vi "FPGA UART.vi"(0 "Clock Frequency":u32=120000000, 1 "Tx IO":refnum<k21>="IO Module\\TTL Out 2", 2 "Rx IO":refnum<k21>="IO Module\\TTL In 3", 5 "Baud Rate":u32=250000, 7 "Data Bits":u8=8 min=5 max=8 step=1, 9 "Stop Bit":u8=1, 11 "Invert Polarity?":bool=TRUE, 12 "Input Valid?":bool, 13 "Tx Data":u8) -> (4 "Rx Data":u8, 6 "Data Received?":bool, 15 "Ready for Input?":bool)   [LabVIEW 2015]
uses:
  Tick Counts.ctl
  Rx States.ctl
  Tx States.ctl
  <vilib>/rvi/FXPMathLib/FxpDiv/subVIs/nifxpmath_Div_SimConfig.ctl
  <vilib>/rvi/Emulation/niFpgaSctlEmulationGetInTimedLoop.vi
  <vilib>/rvi/Emulation/niFpgaProcessEmulError.vi
  <vilib>/rvi/eio/common/nirviEmuTemplateMethod_errors.vi
  <vilib>/rvi/FXPMathLib/FxpDiv/simVIs/DllFxpDivTemp_sub.vi
  <vilib>/eio/EIONode/EIONode.xnode
  <vilib>/rvi/FXPMathLib/FxpDiv/XNode/nifxpmath_Div.xnode
panel:
  out "Tick Counts":T1
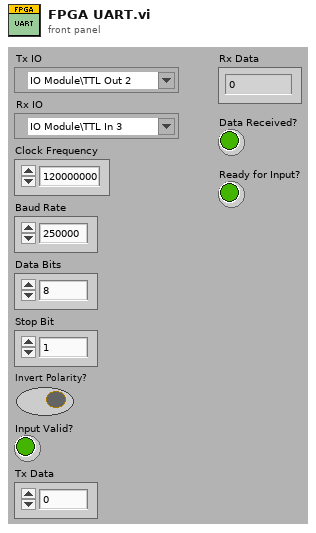
[diagram p1: front panel]
types:
  T1 = typedef "Tick Counts.ctl" = cluster{"Half Bit":u32, "One Bit":u32, "One and Half Bit":u32, "Two Bit":u32}
  T2 = typedef "Tx States.ctl" = enum16{"Wait for Input", "Send Start Bit", "Wait Start", "Send Data Bits", "Wait Send", "Send Parity Bit", "Wait Parity", "Send Stop Bit", "Wait 1 Bit", "Wait 1.5 Bit", "Wait 2 Bit"}
  T3 = typedef "Rx States.ctl" = enum16{"Wait for Start", "Wait Start", "Wait Receive", "Receive Data Bits", "Receive Parity Bit", "Wait Parity", "Wait 1 Bit", "Wait 1.5 Bit", "Wait 2 Bit", "Transfer Rx Data"}
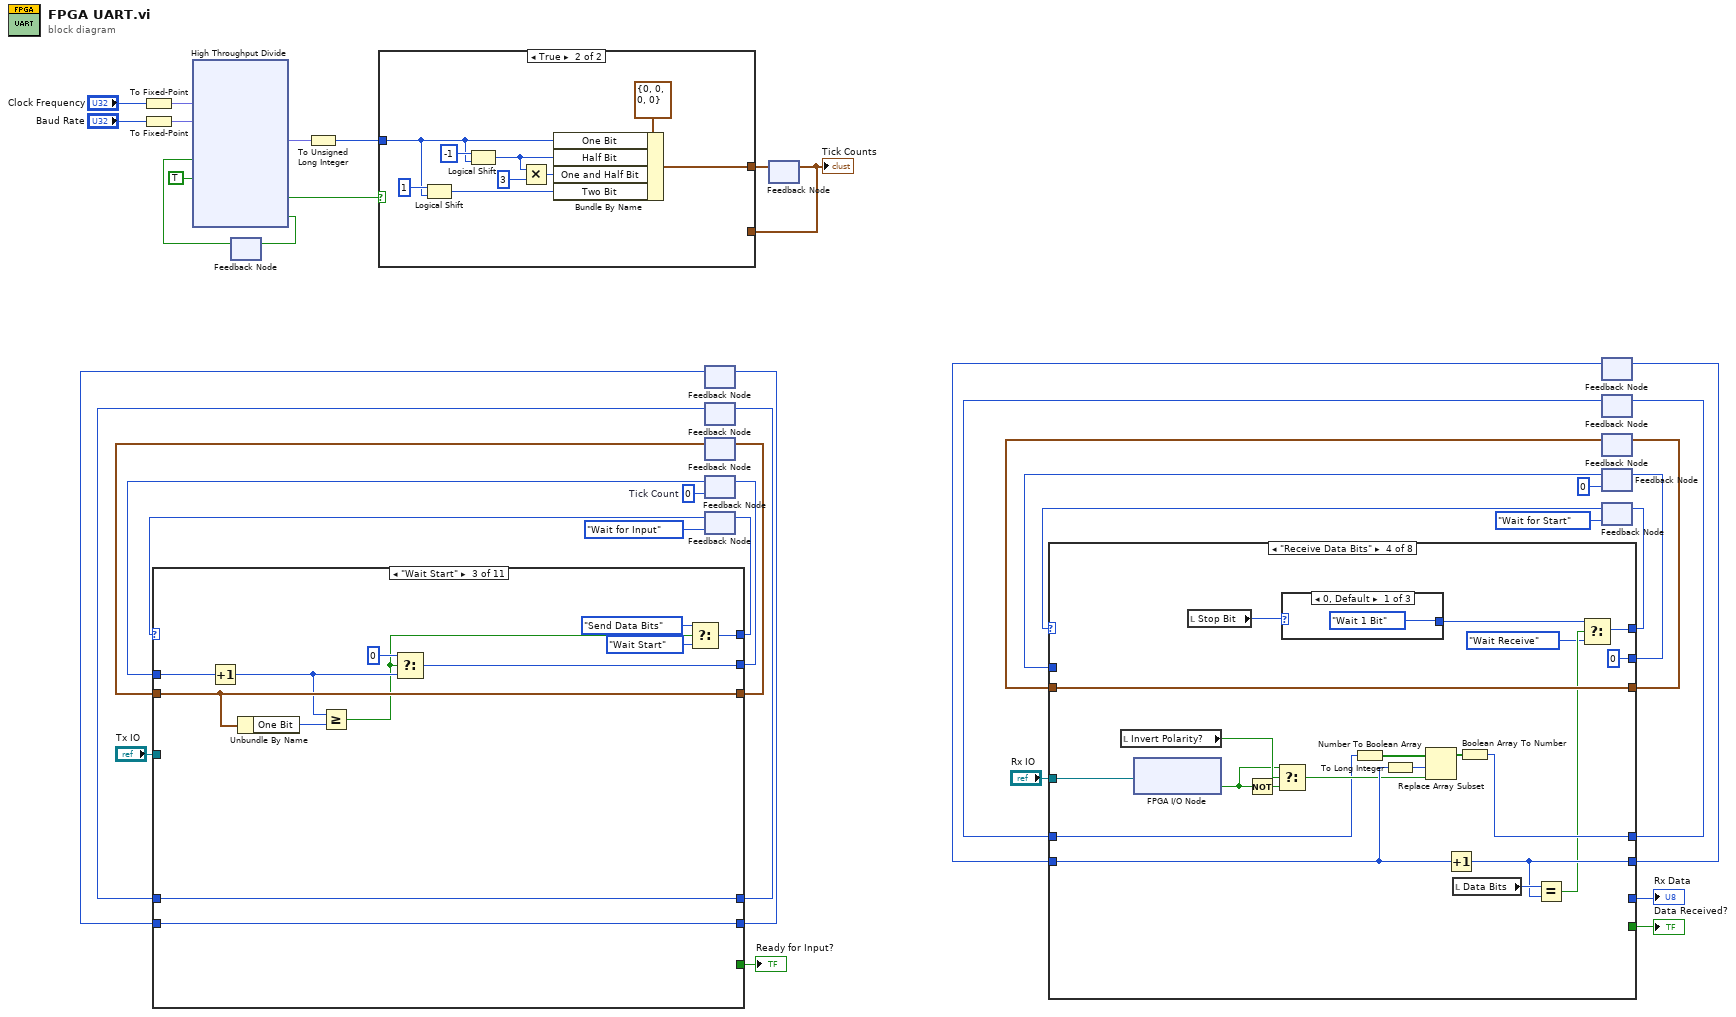
[diagram p0: block diagram]
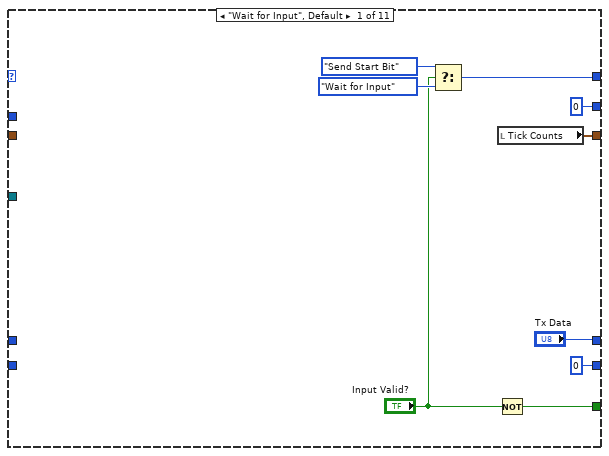
[diagram p2: hidden frame]
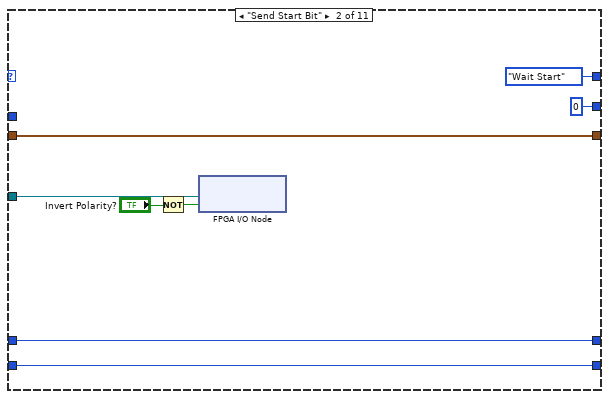
[diagram p3: hidden frame]
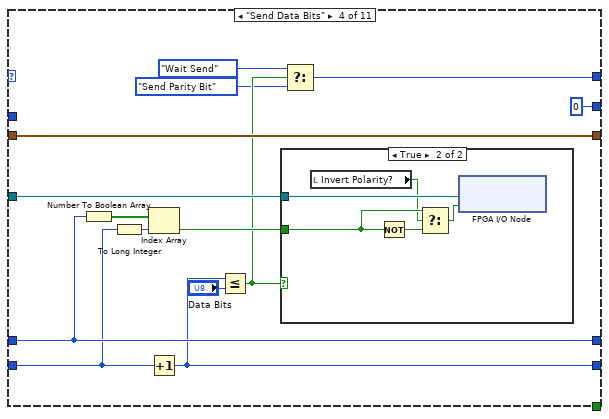
[diagram p4: hidden frame]
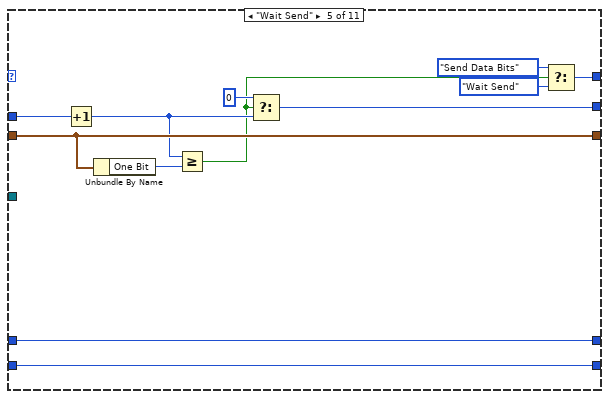
[diagram p6: hidden frame]
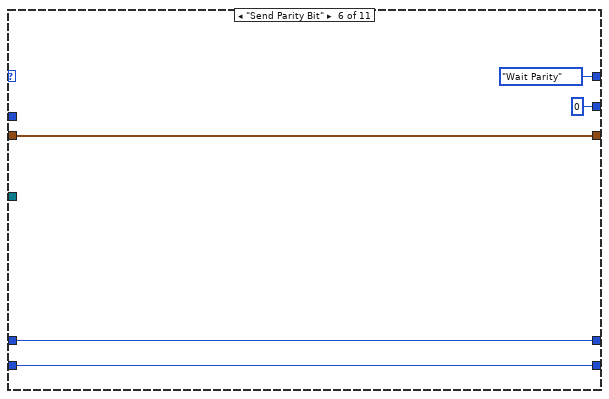
[diagram p7: hidden frame]
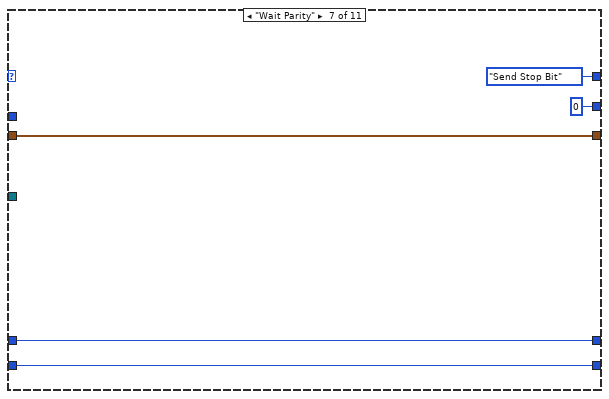
[diagram p8: hidden frame]
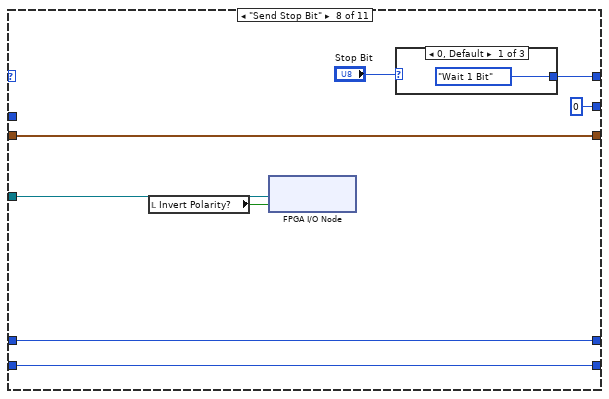
[diagram p9: hidden frame]
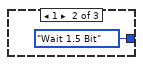
[diagram p10: hidden frame]
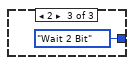
[diagram p11: hidden frame]
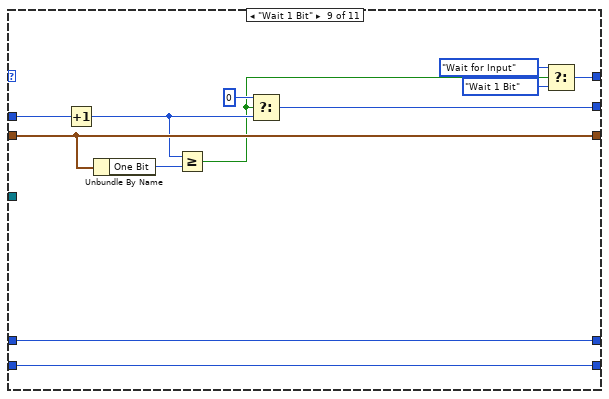
[diagram p12: hidden frame]
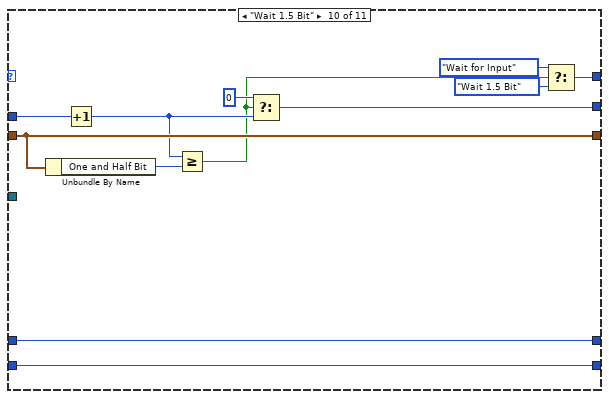
[diagram p13: hidden frame]
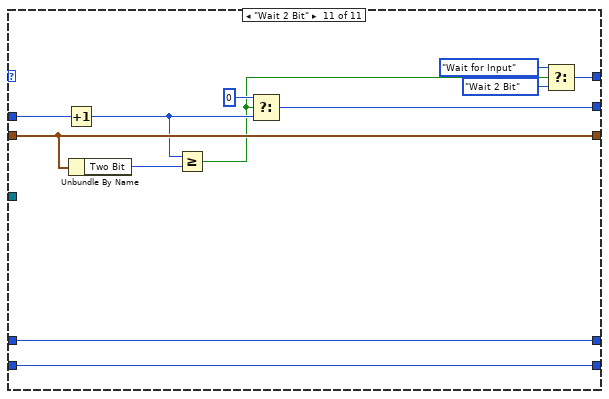
[diagram p14: hidden frame]
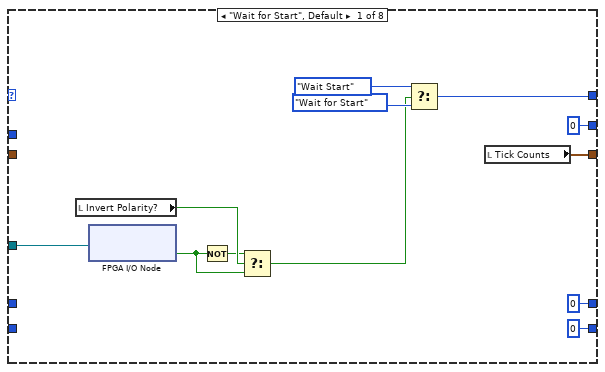
[diagram p15: hidden frame]
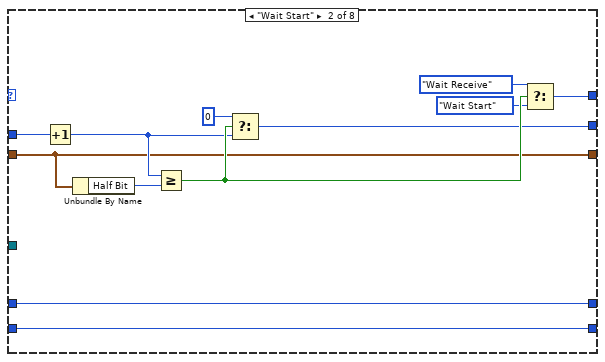
[diagram p16: hidden frame]
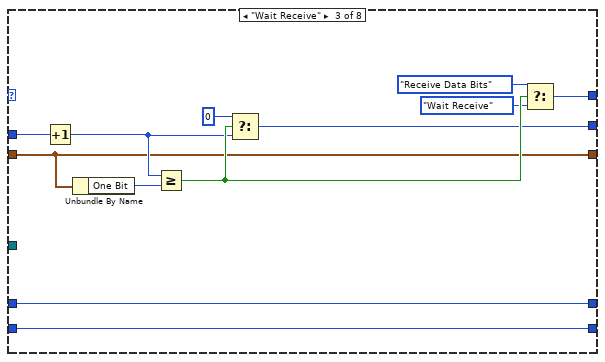
[diagram p17: hidden frame]
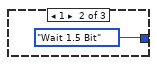
[diagram p18: hidden frame]
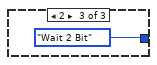
[diagram p19: hidden frame]
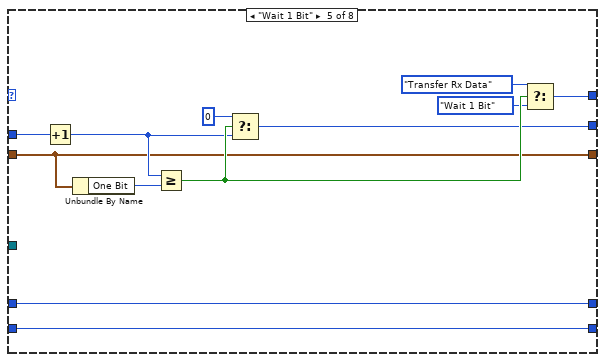
[diagram p20: hidden frame]
diagram:
  w9 = u32 0  # Tick Count
  n1 = To Fixed-Point(number="Clock Frequency") -> (fixed-point=w39:fxp<+,32,32>)  [unwired: 1 in]
  n2 = To Fixed-Point(number="Baud Rate") -> (fixed-point=w38:fxp<+,32,32>)  [unwired: 1 in]
  n3 = feedback #1() -> (w36:bool)  [unwired: 1 in]
  n4 = xnode "High Throughput Divide"("x"=w39, "y"=w38, "input valid"=w36, "ready for output (T)"=TRUE) -> ("x/y"=w33:fxp<+,32,32>, "output valid"=w34:bool, "ready for input"=w37:bool)
  n5 = feedback-in #1(w37) -> ()
  n6 = To Unsigned Long Integer(number=w33) -> (unsigned 32bit integer=w32:u32)
  n7 = feedback #2() -> (w5:u8)  [unwired: 1 in]
  n8 = feedback #3() -> (w7:u8)  [unwired: 1 in]
  n9 = feedback #4() -> (w4:T1)  [unwired: 1 in]
  n10 = feedback #5(w9) -> (w10:u32)
  n11 = feedback #6(Tx_States."Wait for Input" ("Enum")) -> (w13:T2)
  n12 = case shown="\"Wait Start\"" w13 {
    tunnel: [w45 Tx_States."Wait Start" ("Enum") w64 w73 w95 Tx_States."Wait Parity" ("Enum") Tx_States."Send Stop Bit" ("Enum") w113 w128 w140 w152] -> w14
    tunnel: ["Tx Data" w56 w60 w83 w91 w103 w107 w115 w124 w136 w148] -> w3
    tunnel: w7 -> [_ w56 w60 w83 w91 w103 w107 w115 w124 w136 w148]
    tunnel: "Tx IO" -> [_ w58 _ w76 _ _ _ w116 _ _ _]
    tunnel: w10 -> [_ _ w70 _ w101 _ _ _ w134 w146 w158]
    tunnel: [u32 0 u32 0 ("t") w66 u32 0 ("t") w97 u32 0 ("t") u32 0 ("t") u32 0 ("t") w130 w142 w154] -> w11
    tunnel: [w44 w54 w69 w81 w100 w106 w111 w119 w133 w145 w157] -> w8
    tunnel: w4 -> [_ w54 w69 w81 w100 w106 w111 w119 w133 w145 w157]
    tunnel: w5 -> [_ w52 w59 w80 w90 w105 w110 w118 w123 w135 w147]
    tunnel: [u8 0 ("Send Bit Count") w52 w59 w78 w90 w105 w110 w118 w123 w135 w147] -> w6
    tunnel: [w42 _ _ _ _ _ _ _ _ _ _] -> w2
    frame "Wait for Input", Default {
      n13 = Select(t=Tx_States."Send Start Bit", s="Input Valid?", f=Tx_States."Wait for Input" ("Enum")) -> (s? t:f=w45:T2)
      n14 = Not(x="Input Valid?") -> (.not. x?=w42:bool)
      n15 = local read "Tick Counts"() -> (w44:T1)
    }
    frame "Send Start Bit" {
      n16 = Not(x="Invert Polarity?") -> (.not. x?=w57:bool)
      n17 = xnode "FPGA I/O Node"("I/O Item"=w57, "FPGA I/O In"=w58) -> ()  [unwired: 1 out]
    }
    frame "Wait Start" {
      n18 = Increment(x=w70) -> (x+1=w67:u32)
      n19 = Unbundle By Name(w69) -> ("One Bit"=w68:u32)
      n20 = Greater Or Equal?(x=w67, y=w68) -> (x >= y?=w63:bool)
      n21 = Select(t=u32 0, s=w63, f=w67) -> (s? t:f=w66:u32)
      n22 = Select(t=Tx_States."Send Data Bits", s=w63, f=Tx_States."Wait Start" ("Enum")) -> (s? t:f=w64:T2)
    }
    frame "Send Data Bits" {
      n23 = Number To Boolean Array(number=w83) -> (Boolean array=w82:bool[])
      n24 = To Long Integer(number=w80) -> (32bit integer=w79:i32)
      n25 = Index Array(array=w82, index=w79) -> (element=w75:bool)
      n26 = Increment(x=w80) -> (x+1=w78:u8)
      n27 = Less Or Equal?(x=w78, y="Data Bits") -> (x <= y?=w72:bool)
      n28 = case shown="True" w72 {
        tunnel: w76 -> [_ w89]
        tunnel: w75 -> [_ w88]
        frame False {
        }
        frame True {
          n29 = local read "Invert Polarity?"() -> (w85:bool)
          n30 = Not(x=w88) -> (.not. x?=w87:bool)
          n31 = Select(t=w88, s=w85, f=w87) -> (s? t:f=w86:bool)
          n32 = xnode "FPGA I/O Node"("I/O Item"=w86, "FPGA I/O In"=w89) -> ()  [unwired: 1 out]
        }
      }
      n33 = Select(t=Tx_States."Wait Send" ("Enum"), s=w72, f=Tx_States."Send Parity Bit") -> (s? t:f=w73:T2)
    }
    frame "Wait Send" {
      n34 = Increment(x=w101) -> (x+1=w98:u32)
      n35 = Unbundle By Name(w100) -> ("One Bit"=w99:u32)
      n36 = Greater Or Equal?(x=w98, y=w99) -> (x >= y?=w94:bool)
      n37 = Select(t=u32 0, s=w94, f=w98) -> (s? t:f=w97:u32)
      n38 = Select(t=Tx_States."Send Data Bits", s=w94, f=Tx_States."Wait Send" ("Enum")) -> (s? t:f=w95:T2)
    }
    frame "Send Parity Bit" {
    }
    frame "Wait Parity" {
    }
    frame "Send Stop Bit" {
      n39 = local read "Invert Polarity?"() -> (w117:bool)
      n40 = xnode "FPGA I/O Node"("I/O Item"=w117, "FPGA I/O In"=w116) -> ()  [unwired: 1 out]
      n41 = case shown="0, Default" "Stop Bit" {
        tunnel: [Tx_States."Wait 1 Bit" ("Enum") Tx_States."Wait 1.5 Bit" ("Enum") Tx_States."Wait 2 Bit" ("Enum")] -> w113
        frame 0, Default {
        }
        frame 1 {
        }
        frame 2 {
        }
      }
    }
    frame "Wait 1 Bit" {
      n42 = Increment(x=w134) -> (x+1=w131:u32)
      n43 = Unbundle By Name(w133) -> ("One Bit"=w132:u32)
      n44 = Greater Or Equal?(x=w131, y=w132) -> (x >= y?=w127:bool)
      n45 = Select(t=u32 0, s=w127, f=w131) -> (s? t:f=w130:u32)
      n46 = Select(t=Tx_States."Wait for Input", s=w127, f=Tx_States."Wait 1 Bit" ("Enum")) -> (s? t:f=w128:T2)
    }
    frame "Wait 1.5 Bit" {
      n47 = Unbundle By Name(w145) -> ("One and Half Bit"=w144:u32)
      n48 = Increment(x=w146) -> (x+1=w143:u32)
      n49 = Greater Or Equal?(x=w143, y=w144) -> (x >= y?=w139:bool)
      n50 = Select(t=u32 0, s=w139, f=w143) -> (s? t:f=w142:u32)
      n51 = Select(t=Tx_States."Wait for Input", s=w139, f=Tx_States."Wait 1.5 Bit" ("Enum")) -> (s? t:f=w140:T2)
    }
    frame "Wait 2 Bit" {
      n52 = Increment(x=w158) -> (x+1=w155:u32)
      n53 = Unbundle By Name(w157) -> ("Two Bit"=w156:u32)
      n54 = Greater Or Equal?(x=w155, y=w156) -> (x >= y?=w151:bool)
      n55 = Select(t=u32 0, s=w151, f=w155) -> (s? t:f=w154:u32)
      n56 = Select(t=Tx_States."Wait for Input", s=w151, f=Tx_States."Wait 2 Bit" ("Enum")) -> (s? t:f=w152:T2)
    }
  }
  "Ready for Input?" <- w2
  n57 = feedback-in #2(w6) -> ()
  n58 = feedback-in #3(w3) -> ()
  n59 = feedback-in #4(w8) -> ()
  n60 = feedback-in #5(w11) -> ()
  n61 = feedback-in #6(w14) -> ()
  n62 = feedback #7() -> (w16:T1)  [unwired: 1 in]
  "Tick Counts" <- w16
  n63 = case shown="True" w34 {
    tunnel: w32 -> [_ w161]
    tunnel: [w159 w160] -> w17
    tunnel: w16 -> [w159 _]
    frame False {
    }
    frame True {
      n64 = Logical Shift(y=i16 1, x=w161) -> (x << y=w162:u32)
      n65 = Logical Shift(y=i16 -1, x=w161) -> (x << y=w164:u32)
      n66 = Multiply(x=w164, y=u32 3) -> (x*y=w165:u32)
      n67 = Bundle By Name(cluster=T1 {"Half Bit"=0, "One Bit"=0, "One and Half Bit"=0, "Two Bit"=0}, "One Bit"=w161, "Half Bit"=w164, "One and Half Bit"=w165, "Two Bit"=w162) -> (w160:T1)
    }
  }
  n68 = feedback-in #7(w17) -> ()
  n69 = feedback #8() -> (w19:u8)  [unwired: 1 in]
  n70 = feedback #9() -> (w21:u8)  [unwired: 1 in]
  n71 = feedback #10() -> (w24:T1)  [unwired: 1 in]
  n72 = feedback #11(u32 0 ("t")) -> (w26:u32)
  n73 = feedback #12(Rx_States."Wait for Start" ("Enum")) -> (w29:T3)
  n74 = case shown="\"Receive Data Bits\"" w29 {
    tunnel: [u32 0 w186 w198 u32 0 ("t") w233 w245 w257 u32 0 ("t")] -> w27
    tunnel: [w171 w188 w200 w224 w235 w247 w259 w269] -> w25
    tunnel: [w175 w183 w195 w213 w230 w242 w254 Rx_States."Wait for Start" ("Enum")] -> w30
    tunnel: w24 -> [_ w188 w200 w224 w235 w247 w259 w269]
    tunnel: "Rx IO" -> [w170 _ _ w205 _ _ _ _]
    tunnel: w26 -> [_ w187 w199 _ w234 w246 w258 _]
    tunnel: w19 -> [_ w182 w194 w220 w229 w241 w253 w268]
    tunnel: [u8 0 w182 w194 w211 w229 w241 w253 w268] -> w20
    tunnel: w21 -> [_ w181 w193 w216 w228 w240 w252 w265]
    tunnel: [u8 0 ("Rx Data") w181 w193 w214 w228 w240 w252 w265] -> w22
    tunnel: [_ _ _ _ _ _ _ w265] -> w18
    tunnel: [_ _ _ _ _ _ _ TRUE] -> w1
    frame "Wait for Start", Default {
      n75 = local read "Invert Polarity?"() -> (w180:bool)
      n76 = xnode "FPGA I/O Node"("FPGA I/O In"=w170) -> ("I/O Item"=w169:bool)  [unwired: 1 out]
      n77 = Not(x=w169) -> (.not. x?=w179:bool)
      n78 = Select(t=w179, s=w180, f=w169) -> (s? t:f=w176:bool)
      n79 = Select(t=Rx_States."Wait Start" ("Enum"), s=w176, f=Rx_States."Wait for Start" ("Enum")) -> (s? t:f=w175:T3)
      n80 = local read "Tick Counts"() -> (w171:T1)
    }
    frame "Wait Start" {
      n81 = Increment(x=w187) -> (x+1=w190:u32)
      n82 = Unbundle By Name(w188) -> ("Half Bit"=w189:u32)
      n83 = Greater Or Equal?(x=w190, y=w189) -> (x >= y?=w192:bool)
      n84 = Select(t=u32 0, s=w192, f=w190) -> (s? t:f=w186:u32)
      n85 = Select(t=Rx_States."Wait Receive" ("Enum"), s=w192, f=Rx_States."Wait Start" ("Enum")) -> (s? t:f=w183:T3)
    }
    frame "Wait Receive" {
      n86 = Increment(x=w199) -> (x+1=w202:u32)
      n87 = Unbundle By Name(w200) -> ("One Bit"=w201:u32)
      n88 = Greater Or Equal?(x=w202, y=w201) -> (x >= y?=w204:bool)
      n89 = Select(t=u32 0, s=w204, f=w202) -> (s? t:f=w198:u32)
      n90 = Select(t=Rx_States."Receive Data Bits" ("Enum"), s=w204, f=Rx_States."Wait Receive" ("Enum")) -> (s? t:f=w195:T3)
    }
    frame "Receive Data Bits" {
      n91 = local read "Invert Polarity?"() -> (w223:bool)
      n92 = xnode "FPGA I/O Node"("FPGA I/O In"=w205) -> ("I/O Item"=w222:bool)  [unwired: 1 out]
      n93 = local read "Stop Bit"() -> (w207:u8)
      n94 = Not(x=w222) -> (.not. x?=w221:bool)
      n95 = Select(t=w222, s=w223, f=w221) -> (s? t:f=w218:bool)
      n96 = case shown="0, Default" w207 {
        tunnel: [Rx_States."Wait 1 Bit" ("Enum") Rx_States."Wait 1.5 Bit" ("Enum") Rx_States."Wait 2 Bit" ("Enum")] -> w206
        frame 0, Default {
        }
        frame 1 {
        }
        frame 2 {
        }
      }
      n97 = Number To Boolean Array(number=w216) -> (Boolean array=w217:bool[])
      n98 = To Long Integer(number=w220) -> (32bit integer=w219:i32)
      n99 = Replace Array Subset(array=w217, new element=w218, index=w219) -> (w215:bool[])
      n100 = Increment(x=w220) -> (x+1=w211:u8)
      n101 = local read "Data Bits"() -> (w212:u8)
      n102 = Boolean Array To Number(Boolean array=w215) -> (number=w214:u8)
      n103 = Equal?(x=w212, y=w211) -> (x = y?=w210:bool)
      n104 = Select(t=w206, s=w210, f=Rx_States."Wait Receive" ("Enum")) -> (s? t:f=w213:T3)
    }
    frame "Wait 1 Bit" {
      n105 = Increment(x=w234) -> (x+1=w237:u32)
      n106 = Unbundle By Name(w235) -> ("One Bit"=w236:u32)
      n107 = Greater Or Equal?(x=w237, y=w236) -> (x >= y?=w239:bool)
      n108 = Select(t=u32 0, s=w239, f=w237) -> (s? t:f=w233:u32)
      n109 = Select(t=Rx_States."Transfer Rx Data" ("Enum"), s=w239, f=Rx_States."Wait 1 Bit" ("Enum")) -> (s? t:f=w230:T3)
    }
    frame "Wait 1.5 Bit" {
      n110 = Unbundle By Name(w247) -> ("One and Half Bit"=w248:u32)
      n111 = Increment(x=w246) -> (x+1=w249:u32)
      n112 = Greater Or Equal?(x=w249, y=w248) -> (x >= y?=w251:bool)
      n113 = Select(t=u32 0, s=w251, f=w249) -> (s? t:f=w245:u32)
      n114 = Select(t=Rx_States."Transfer Rx Data" ("Enum"), s=w251, f=Rx_States."Wait 1.5 Bit" ("Enum")) -> (s? t:f=w242:T3)
    }
    frame "Wait 2 Bit" {
      n115 = Increment(x=w258) -> (x+1=w261:u32)
      n116 = Unbundle By Name(w259) -> ("Two Bit"=w260:u32)
      n117 = Greater Or Equal?(x=w261, y=w260) -> (x >= y?=w263:bool)
      n118 = Select(t=u32 0, s=w263, f=w261) -> (s? t:f=w257:u32)
      n119 = Select(t=Rx_States."Transfer Rx Data" ("Enum"), s=w263, f=Rx_States."Wait 2 Bit" ("Enum")) -> (s? t:f=w254:T3)
    }
    frame "Transfer Rx Data" {
    }
  }
  "Rx Data" <- w18
  "Data Received?" <- w1
  n120 = feedback-in #8(w20) -> ()
  n121 = feedback-in #9(w22) -> ()
  n122 = feedback-in #10(w25) -> ()
  n123 = feedback-in #11(w27) -> ()
  n124 = feedback-in #12(w30) -> ()
